vi "Finish.vi"   [LabVIEW 2012]
doc: "This VI is called just before exiting. It is expected to close I/O refnum, save collected data, etc."
uses:
  <vilib>/Rock Robotics/WPI/Compressor/WPI_CompressorGetSetRefNum.vi
  <vilib>/Rock Robotics/WPI/Joystick/WPI_JoystickGetSetRefNum.vi
  <vilib>/Rock Robotics/WPI/RobotDrive/WPI_RobotDriveGetSetRefNum.vi
  F:/Team 1699 2013 robot code/Team 1699 2013 Robot Project V1a/Robot Global Data.vi
  <vilib>/Utility/config.llb/Write Key (Double).vi
  <vilib>/Utility/config.llb/NI_LVConfig.lvlib
types:
  T1 = typedef "NI_LVConfig.lvlib/Config Data RefNum.ctl" = refnum<k1>
  T2 = typedef "WPI_JoystickDevRef.ctl" = cluster{"Device":T3}
  T3 = typedef "WPI_JoystickDeviceEnum.ctl" = enum16{"USB 1", "USB 2", "USB 3", "USB 4", "Kinect 1", "Kinect 2"}
  T4 = typedef "WPI_RobotDriveDevRef.ctl" = cluster{"DevStatus":errorcluster, "Motors[]":T5[], "Square Inputs":bool, "Max Output":dbl, "Isochronous":bool}
  T5 = typedef "WPI_MotorControlDeviceRef.ctl" = cluster{"DeviceStatus":errorcluster, "Type":enum16{"PWM", "CAN"}, "PWM":cluster{"Digital Module":T6, "PWM Channel":T7, "DeadBand":T8}, "CAN":cluster{"Device Number":u8, "Control Mode":T9, "Semaphore":T10, "Max Vout":dbl}, "Invert":bool, "TransformRef":T11, "InvTransformRef":T11}
  T6 = typedef "FPGA_TypedefDigitalModule.ctl" = enum16{"Digital Module 1", "Digital Module 2"}
  T7 = typedef "FPGA_DIOPWMChannel.ctl" = enum8{"PWM 1", "PWM 2", "PWM 3", "PWM 4", "PWM 5", "PWM 6", "PWM 7", "PWM 8", "PWM 9", "PWM 10", "Invalid"}
  T8 = typedef "WPI_PWMDeadband.ctl" = cluster{"Name":string, "maxPositivePwm":i32, "minPositivePwm":i32, "centerPwm":i32, "maxNegativePwm":i32, "minNegativePwm":i32, "angularRange":u16}
  T9 = typedef "WPI_CANJaguar_ControlMode.ctl" = enum8{"Percent VBus", "Current", "Speed", "Position", "Voltage"}
  T10 = typedef "Semaphore RefNum" = refnum<k1>
  T11 = typedef "WPI_PWMTransform_ConPane.ctl" = refnum<vi>
  T12 = typedef "WPI_CameraDevRef.ctl" = cluster{"Camera Address":string, "CameraStatus":errorcluster, "Acquire Image Notifier":refnum<notifier>}
  T13 = typedef "WPI_CompressorDevRef.ctl" = cluster{"DevStatus":errorcluster, "DigitalInputDevRef":T14, "RelayDevRef":T16}
  T14 = typedef "WPI_DigitalInputDevRef.ctl" = cluster{"DevStatus":errorcluster, "DIO Channel":T15, "Digital Module":T6}
  T15 = typedef "FPGA_DIOChannel.ctl" = enum8{"DIO 1", "DIO 2", "DIO 3", "DIO 4", "DIO 5", "DIO 6", "DIO 7", "DIO 8", "DIO 9", "DIO 10", "DIO 11", "DIO 12", "DIO 13", "DIO 14", "Invalid"}
  T16 = typedef "WPI_RelayDevRef.ctl" = cluster{"DevStatus":errorcluster, "Relay Channel":T17, "Digital Module":T6, "Relay Direction":T18}
  T17 = typedef "FPGA_DIORelayChannel.ctl" = enum8{"Relay 1", "Relay 2", "Relay 3", "Relay 4", "Relay 5", "Relay 6", "Relay 7", "Relay 8", "Invalid"}
  T18 = typedef "WPI_RelayDirection.ctl" = enum16{"Both directions", "Forward only", "Reverse only"}
  T19 = typedef "WPI_EncoderDevRef.ctl" = cluster{"DevStatus":errorcluster, "EncoderIndex":T20, "CounterIndex":T21, "DistancePerCount":dbl, "Decoding Type":T22}
  T20 = typedef "FPGA_EncoderIdx.ctl" = enum8{"Enc 0", "Enc 1", "Enc 2", "Enc 3", "Invalid"}
  T21 = typedef "FPGA_CounterCtrSystemIndex.ctl" = enum8{"Ctr 0", "Ctr 1", "Ctr 2", "Ctr 3", "Ctr 4", "Ctr 5", "Ctr 6", "Ctr 7", "Invalid"}
  T22 = typedef "WPI_EncoderType.ctl" = enum16{"1x", "2x", "4x"}
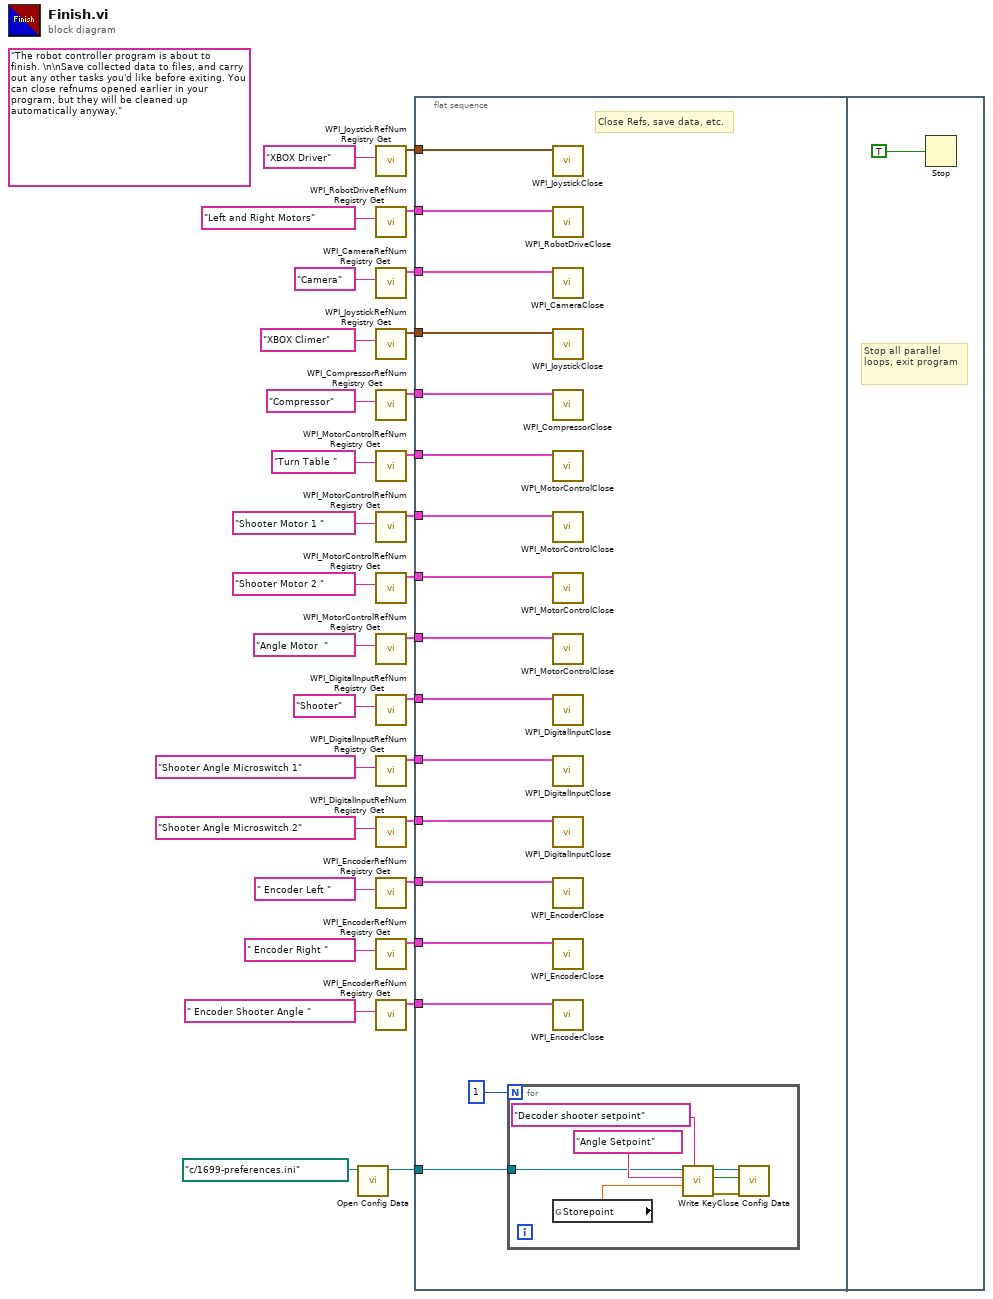
[diagram p0: block diagram]
diagram:
  (unwired) "The robot controller program is about to finish. \n\nSave collected data to files, and carry out any other tasks you'd like before exiting. You can close refnums opened earlier in your program, but they will be cleaned up automatically anyway."
  n1 = call <vilib>:"Open Config Data.vi"("configuration file path"=path "c:/1699-preferences.ini") -> ("refnum"=w1:T1)  [unwired: 8 in, 2 out]
  n2 = call <vilib>:"WPI_JoystickRefNum Registry Get.vi"("refnum name"="XBOX Driver") -> ("JoystickDevRef"=w29:T2)  [unwired: 1 in, 9 out]
  n3 = call <vilib>:"WPI_RobotDriveRefNum Registry Get.vi"("refnum name"="Left and Right Motors") -> ("RobotDriveDevRef"=w30:T4)  [unwired: 1 in, 9 out]
  n4 = call <vilib>:"WPI_CameraRefNum Registry Get.vi"("refnum name"="Camera") -> ("CameraDevRef"=w28:T12)  [unwired: 1 in, 9 out]
  n5 = call <vilib>:"WPI_JoystickRefNum Registry Get.vi"("refnum name"="XBOX Climer") -> ("JoystickDevRef"=w26:T2)  [unwired: 1 in, 9 out]
  n6 = call <vilib>:"WPI_CompressorRefNum Registry Get.vi"("refnum name"="Compressor") -> ("CompressorDevRef"=w24:T13)  [unwired: 9 in, 1 out]
  n7 = call <vilib>:"WPI_MotorControlRefNum Registry Get.vi"("refnum name"="Turn Table ") -> ("MotorControlDevRef"=w22:T5)  [unwired: 9 in, 1 out]
  n8 = call <vilib>:"WPI_MotorControlRefNum Registry Get.vi"("refnum name"="Shooter Motor 1 ") -> ("MotorControlDevRef"=w21:T5)  [unwired: 9 in, 1 out]
  n9 = call <vilib>:"WPI_MotorControlRefNum Registry Get.vi"("refnum name"="Shooter Motor 2 ") -> ("MotorControlDevRef"=w20:T5)  [unwired: 9 in, 1 out]
  n10 = call <vilib>:"WPI_MotorControlRefNum Registry Get.vi"("refnum name"="Angle Motor  ") -> ("MotorControlDevRef"=w19:T5)  [unwired: 9 in, 1 out]
  n11 = call <vilib>:"WPI_DigitalInputRefNum Registry Get.vi"("refnum name"="Shooter") -> ("DigitalInputDevRef"=w14:T14)  [unwired: 9 in, 1 out]
  n12 = call <vilib>:"WPI_DigitalInputRefNum Registry Get.vi"("refnum name"="Shooter Angle Microswitch 1") -> ("DigitalInputDevRef"=w13:T14)  [unwired: 9 in, 1 out]
  n13 = call <vilib>:"WPI_DigitalInputRefNum Registry Get.vi"("refnum name"="Shooter Angle Microswitch 2") -> ("DigitalInputDevRef"=w12:T14)  [unwired: 9 in, 1 out]
  n14 = call <vilib>:"WPI_EncoderRefNum Registry Get.vi"("refnum name"=" Encoder Left ") -> ("EncoderDevRef"=w11:T19)  [unwired: 9 in, 1 out]
  n15 = call <vilib>:"WPI_EncoderRefNum Registry Get.vi"("refnum name"=" Encoder Right ") -> ("EncoderDevRef"=w10:T19)  [unwired: 9 in, 1 out]
  n16 = call <vilib>:"WPI_EncoderRefNum Registry Get.vi"("refnum name"=" Encoder Shooter Angle ") -> ("EncoderDevRef"=w9:T19)  [unwired: 9 in, 1 out]
  n17 = flat-sequence {
    tunnel: w30 -> [w49]
    tunnel: w29 -> [w48]
    tunnel: w28 -> [w47]
    tunnel: w26 -> [w46]
    tunnel: w24 -> [w45]
    tunnel: w22 -> [w44]
    tunnel: w21 -> [w43]
    tunnel: w20 -> [w42]
    tunnel: w19 -> [w41]
    tunnel: w14 -> [w40]
    tunnel: w13 -> [w39]
    tunnel: w12 -> [w38]
    tunnel: w11 -> [w37]
    tunnel: w10 -> [w36]
    tunnel: w9 -> [w35]
    tunnel: w1 -> [w33]
    frame #0 {
      # "Close Refs, save data, etc."
      n18 = for {
        N: 1 -> [_]
        tunnel: w33 -> [w53]
        n19 = global read "Robot Global Data.vi" "Storepoint"() -> (w54:dbl)
        n20 = call-poly <vilib>:"Write Key.vi"("section"="Decoder shooter setpoint", "value"=w54, "key"="Angle Setpoint", "refnum"=w53) -> ("error out"=w52:errorcluster, "found?"=w51:bool, "refnum out"=w50:T1)  [unwired: 5 in]
        n21 = call <vilib>:"Close Config Data.vi"("error in (no error)"=w52, "write file if changed (T)"=w51, "refnum"=w50) -> ()  [unwired: 7 in, 2 out]
      }
      n22 = call <vilib>:"WPI_JoystickClose.vi"("JoystickDevRef"=w48) -> ()  [unwired: 11 out]
      n23 = call <vilib>:"WPI_RobotDriveClose.vi"("RobotDriveDevRef"=w49) -> ()  [unwired: 1 in, 10 out]
      n24 = call <vilib>:"WPI_CameraClose.vi"("CameraDevRef"=w47) -> ()  [unwired: 1 in, 10 out]
      n25 = call <vilib>:"WPI_JoystickClose.vi"("JoystickDevRef"=w46) -> ()  [unwired: 11 out]
      n26 = call <vilib>:"WPI_CompressorClose.vi"("CompressorDevRef"=w45) -> ()  [unwired: 10 in, 1 out]
      n27 = call <vilib>:"WPI_MotorControlClose.vi"("MotorControlDevRef"=w44) -> ()  [unwired: 10 in, 1 out]
      n28 = call <vilib>:"WPI_MotorControlClose.vi"("MotorControlDevRef"=w43) -> ()  [unwired: 10 in, 1 out]
      n29 = call <vilib>:"WPI_MotorControlClose.vi"("MotorControlDevRef"=w42) -> ()  [unwired: 10 in, 1 out]
      n30 = call <vilib>:"WPI_MotorControlClose.vi"("MotorControlDevRef"=w41) -> ()  [unwired: 10 in, 1 out]
      n31 = call <vilib>:"WPI_DigitalInputClose.vi"("DigitalInputDevRef"=w40) -> ()  [unwired: 10 in, 1 out]
      n32 = call <vilib>:"WPI_DigitalInputClose.vi"("DigitalInputDevRef"=w39) -> ()  [unwired: 10 in, 1 out]
      n33 = call <vilib>:"WPI_DigitalInputClose.vi"("DigitalInputDevRef"=w38) -> ()  [unwired: 10 in, 1 out]
      n34 = call <vilib>:"WPI_EncoderClose.vi"("EncoderDevRef"=w37) -> ()  [unwired: 10 in, 1 out]
      n35 = call <vilib>:"WPI_EncoderClose.vi"("EncoderDevRef"=w36) -> ()  [unwired: 10 in, 1 out]
      n36 = call <vilib>:"WPI_EncoderClose.vi"("EncoderDevRef"=w35) -> ()  [unwired: 10 in, 1 out]
    }
    frame #1 {
      # "Stop all parallel\nloops, exit program"
      n37 = Stop(stop? (T)=TRUE ("Quit")) -> ()
    }
  }
